vi "Moons.vi"(8 "error in (no error)":errorcluster caption="entrée d'erreur (pas d'erreur)", 11 "make_moons":T2={"n_samples"="100", "shuffle"=TRUE, "noise"=-1.0, "random_state"=-1, "Returns"="X"} {"noise" min=-1.0; "random_state" min=-1}) -> (0 "error out":errorcluster, 3 "Data":T1)   [LabVIEW 2020]
doc: "Make two interleaving half circles\n\nA simple toy dataset to visualize clustering and classification algorithms. \n\nParameters : \n\n- n_samples : int or two-element tuple, optional (default=100)\nIf int, the total number of points generated. If two-element tuple, number of points in each of two moons.\n\n- shuffle : bool, optional (default=True)\nWhether to shuffle the samples.\n\n- noise : double or None (default=None=-1)\nStandard deviation of Gaussian noise added to the data.\n\n- random_state : int, RandomState instance, default=None=-1\nDetermines random number generation for dataset shuffling and noise. Pass an int for reproducible output across multiple function calls. See Glossary.\n\nReturns :\n\n- X : array of shape [n_samples, 2]\nThe generated samples.\n\n- y : array of shape [n_samples]\nThe integer labels (0 or 1) for class membership of each sample."
uses:
  Moons.lvclass
panel:
  out "Moons.lvclass":refnum<class "Moons.lvclass">
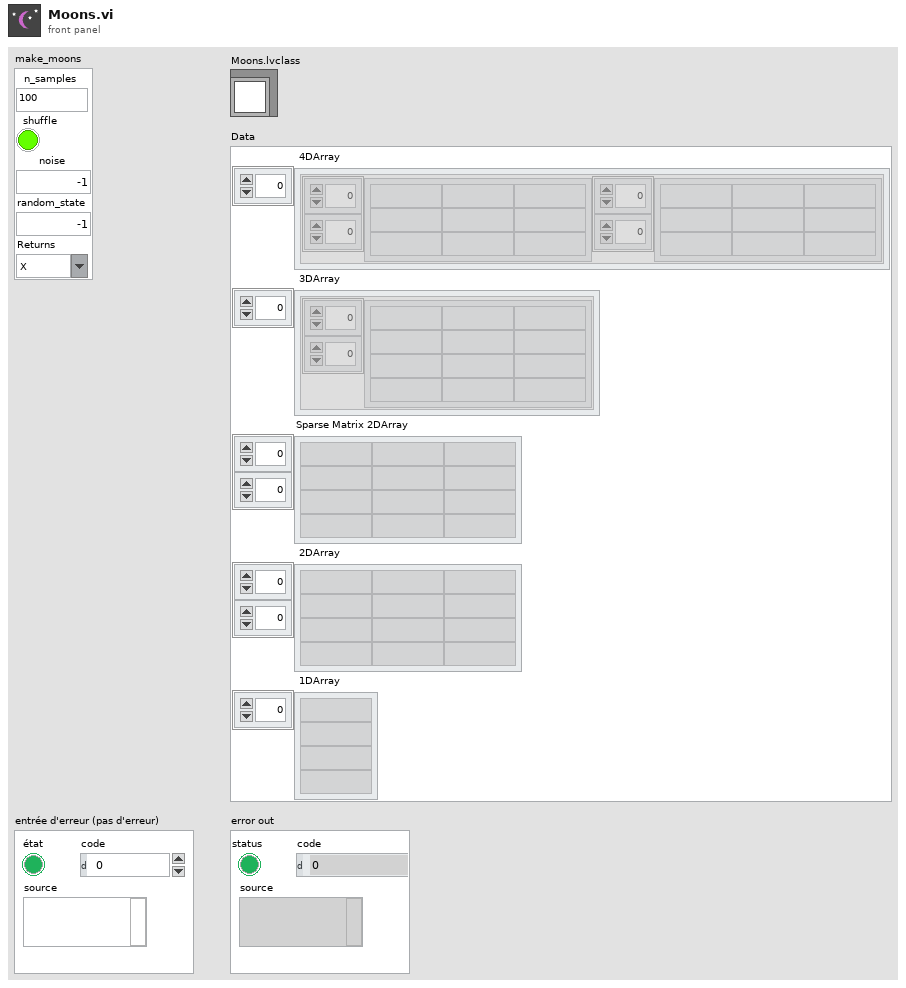
[diagram p1: front panel]
types:
  T1 = cluster{" 4DArray":cluster{"1":string[][], "2":string[][]}[], " 3DArray":cluster{"Tableau":string[][]}[], "Sparse Matrix 2DArray":string[][], " 2DArray":string[][], " 1DArray":string[]}
  T2 = cluster{"n_samples":string, "shuffle":bool, "noise":dbl, "random_state":i32, "Returns":string}
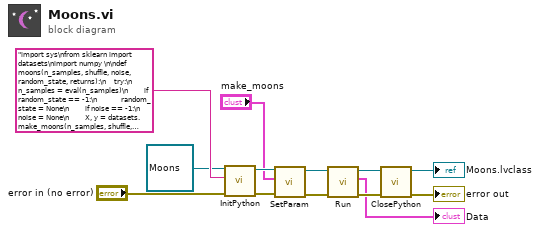
[diagram p0: block diagram]
diagram:
  n1 = call-dynamic "InitPython.vi"("error in (no error)"="error in (no error)", "Python Instruction"="import sys\nfrom sklearn import datasets\nimport numpy \n\ndef moons(n_samples, shuffle, noise, random_state, returns):\n    try:\n        n_samples = eval(n_samples)\n        if random_state == -1:\n            random_state = None\n        if noise == -1:\n            noise = None\n        X, y = datasets.make_moons(n_samples, shuffle, noise, random_state)\n        if returns == 'X':\n            dataX = X.tolist()\n            return str(dataX)\n        else:\n            datay = y.tolist()\n            return str(datay)\n    except:\n        erreur = sys.exc_info()\n        typerr = u\"%s\" % (erreur[0])\n        typerr = typerr[typerr.find(\"'\")+1:typerr.rfind(\"'\")]\n        msgerr = u\"%s\" % (erreur[1])\n        message = str('/!\\\\ {0} : {1}'. format(typerr,msgerr))\n        return message", "Scikit-learn en entrée"=refnum<class "Moons.lvclass"> refnum ("Moons.lvclass")) -> ("error out"=w9:errorcluster, "Scikit-learn en sortie"=w10:refnum<class "Moons.lvclass">)  [unwired: 7 in]
  n2 = call-dynamic "SetParam.vi"("error in (no error)"=w9, "make_moons"="make_moons", "Moons.lvclass"=w10) -> ("error out"=w6:errorcluster, "Moons.lvclass"=w7:refnum<class "Moons.lvclass">)  [unwired: 7 in]
  n3 = call-dynamic "Run.vi"("error in (no error)"=w6, "Moons.lvclass"=w7) -> ("error out"=w4:errorcluster, "Data"=→"Data":T1, "Moons.lvclass"=w5:refnum<class "Moons.lvclass">)  [unwired: 7 in]
  n4 = call-dynamic "ClosePython.vi"("error in (no error)"=w4, "Scikit-learn en entrée"=w5) -> ("error out"=→"error out":errorcluster, "Scikit-learn en sortie"=→"Moons.lvclass":refnum<class "Moons.lvclass">)  [unwired: 8 in]
